vi "Waterfall Page.vi"() -> ()   [LabVIEW 2017, in "3D Waterfall.lvclass"]
uses:
  <vilib>/Math Plots/3D Math Plots/3D Waterfall/3D Waterfall/3D Waterfall.lvclass
  <vilib>/Math Plots/3D Math Plots/3D Waterfall/3D Waterfall/Typedef/3D Waterfall Propery Array.ctl
  <vilib>/Math Plots/3D Math Plots/3D Waterfall/3D Waterfall/Typedef/3D Waterfall Property.ctl
  <vilib>/Math Plots/3D Math Plots/3D Plot/3D Plot/Typedef/Line Type.ctl
  <vilib>/Math Plots/3D Math Plots/3D Plot/3D Plot/Typedef/Color Ramp Cluster.ctl
  <vilib>/Math Plots/3D Math Plots/3D Plot/3D Plot/Typedef/Dialog State.ctl
  <vilib>/Math Plots/3D Math Plots/3D Plot/3D Plot/Typedef/Temp Scene State.ctl
  <vilib>/Math Plots/3D Math Plots/3D Plot/3D Plot/Typedef/Temp Scene Property Action.ctl
  <vilib>/Math Plots/3D Math Plots/3D Plot/3D Plot/3D Plot.lvclass
panel:
  in  "Waterfall Mode":u16(ring) caption="Waterfall mode" items=["Lines", "Slices"]
  in  "Line Style":u16(ring) caption="Line style"
  in  "Antialiasing":bool
  in  "Line Width":sgl=0.001 caption="Line width" min=0.001 step=1
  out "Waterfall Property Out":T1
  in  "Waterfall Property In":T1
  out "Color Ramp":dbl[][](graph)
  in  "Color Map Style":u16(ring) caption="Color map style" items=["None ", "Shaded", "Color spectrum", "Grey scale", "Custom"]
  in  "YZ Plane Projection":bool caption="YZ plane projection"
  in  "XZ Plane Projection":bool caption="XZ plane projection"
  in  "XY Plane Projection":bool caption="XY plane projection"
  in  "Coordinate System":u16(ring) caption="Coordinate system" items=["Cartesian", "Cylindrical", "Spherical"]
  in  "Plot Opacity":sgl(slide) caption="Plot opacity(%)" min=0 max=100 scale=0.0..100.0
  in  "Plot List":i32(listbox)
  in  "Ramp Edit":bool caption="Ramp edit"
  in  "Move Down":bool
  in  "Move Up":bool
  in  "Delete":bool
  in  "New":bool
  in  "Event Registration":refnum<event-registration>
  # "Waterfall"
  # "General"
  # "Projection"
  # "Color Ramp"
  # "Waterfall"
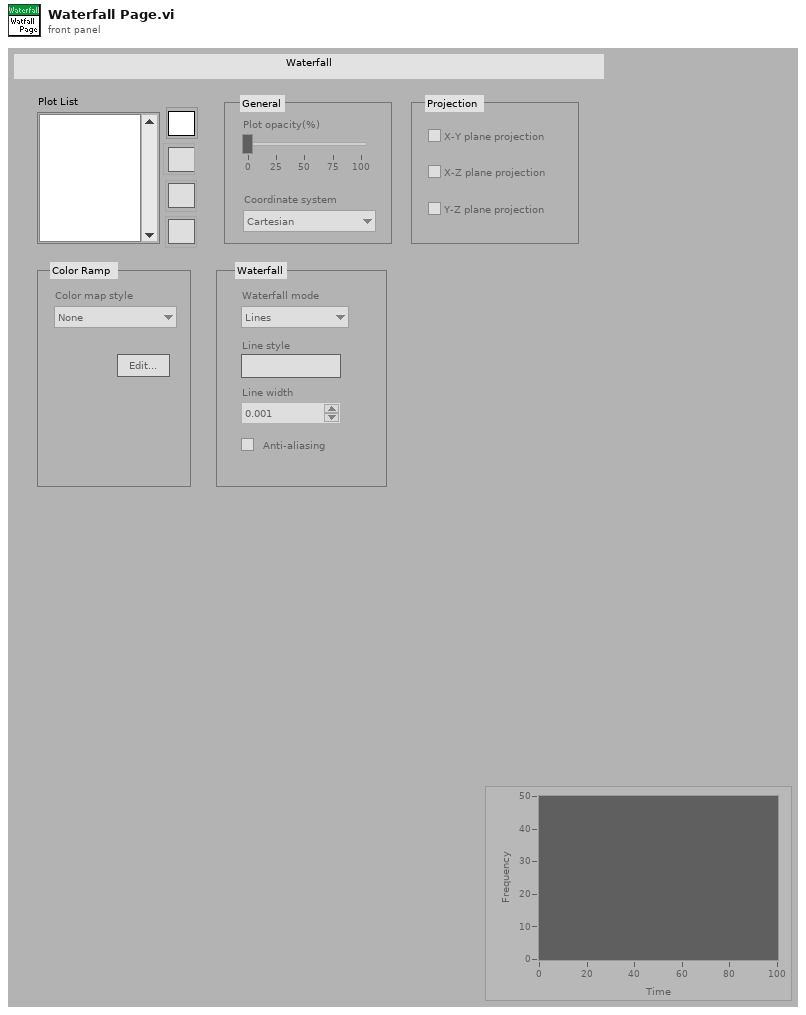
[diagram p1: front panel]
types:
  T1 = typedef "3D Waterfall.lvclass/3D Waterfall Propery Array.ctl" = T2[]
  T2 = typedef "3D Waterfall.lvclass/3D Waterfall Property.ctl" = cluster{"General Property":cluster{"Plot Name":string, "Coordinate System":enum16{"Cartesian", "Cylindrical", "Spherical"}, "Opacity":sgl}, "Projection Property":cluster{"Draw XY":bool, "Draw YZ":bool, "Draw XZ":bool}, "Plot Property":cluster{"Line Style":T3, "Line Width":sgl, "Color Ramp Cluster":T4, "Antialiasing":bool}, "Waterfall Property":cluster{"Waterfall Mode":enum16{"Lines", "Slices"}}}
  T3 = typedef "3D Plot.lvclass/Line Type.ctl" = enum16{"None", "Solid", "Dash", "Dot", "Dash Dot"}
  T4 = typedef "3D Plot.lvclass/Color Ramp Cluster.ctl" = cluster{"Color Ramp Style":enum16{"None", "Shaded", "Color spectrum", "Grey scale", "Custom"}, "Color Ramp Array":u32[], "Color Ramp Index":i32[], "Interpolate?":bool, "Logarithm?":bool}
  T5 = typedef "3D Plot.lvclass/Dialog State.ctl" = enum16{"Initialize", "Read Porperty", "Write Property", "Idle", "Exit"}
  T6 = typedef "3D Plot.lvclass/Temp Scene State.ctl" = enum16{"Create", "Update Scene", "Get Plot Representation", "Destory"}
  T7 = typedef "3D Plot.lvclass/Temp Scene Property Action.ctl" = enum16{"Graph Property", "Light Property", "Axis Property", "Value Pair Property", "Format Property", "Cursor Property", "Plot Specific Property"}
  T8 = typedef "3D Plot.lvclass/Multiplot Representation.ctl" = cluster{"Plot Represention Array":T9[], "Max Range":T10}
  T9 = typedef "3D Plot.lvclass/Plot Representation.ctl" = cluster{"Plot ID":i32, "Plot Range":T10, "Mesh Data":T11, "Dimension":cluster{"X Dimension":i32, "Y Dimension":i32}, "Ramp Range":T10}
  T10 = typedef "3D Plot.lvclass/Range Clusters.ctl" = cluster{"X Range":cluster{"Max X":sgl, "Min X":sgl}, "Y Range":cluster{"Max Y":sgl, "Min Y":sgl}, "Z Range":cluster{"Max Z":sgl, "Min Z":sgl}}
  T11 = typedef "3D Plot.lvclass/Mesh Data.ctl" = cluster{"Index Array":u32[], "Vertex Array":cluster{"X":sgl, "Y":sgl, "Z":sgl}[], "Normal Array":cluster{"X":sgl, "Y":sgl, "Z":sgl}[], "Color Index Array":i32[]}
  T12 = enum16{"None", "Shaded", "Color spectrum", "Grey scale", "Custom"}
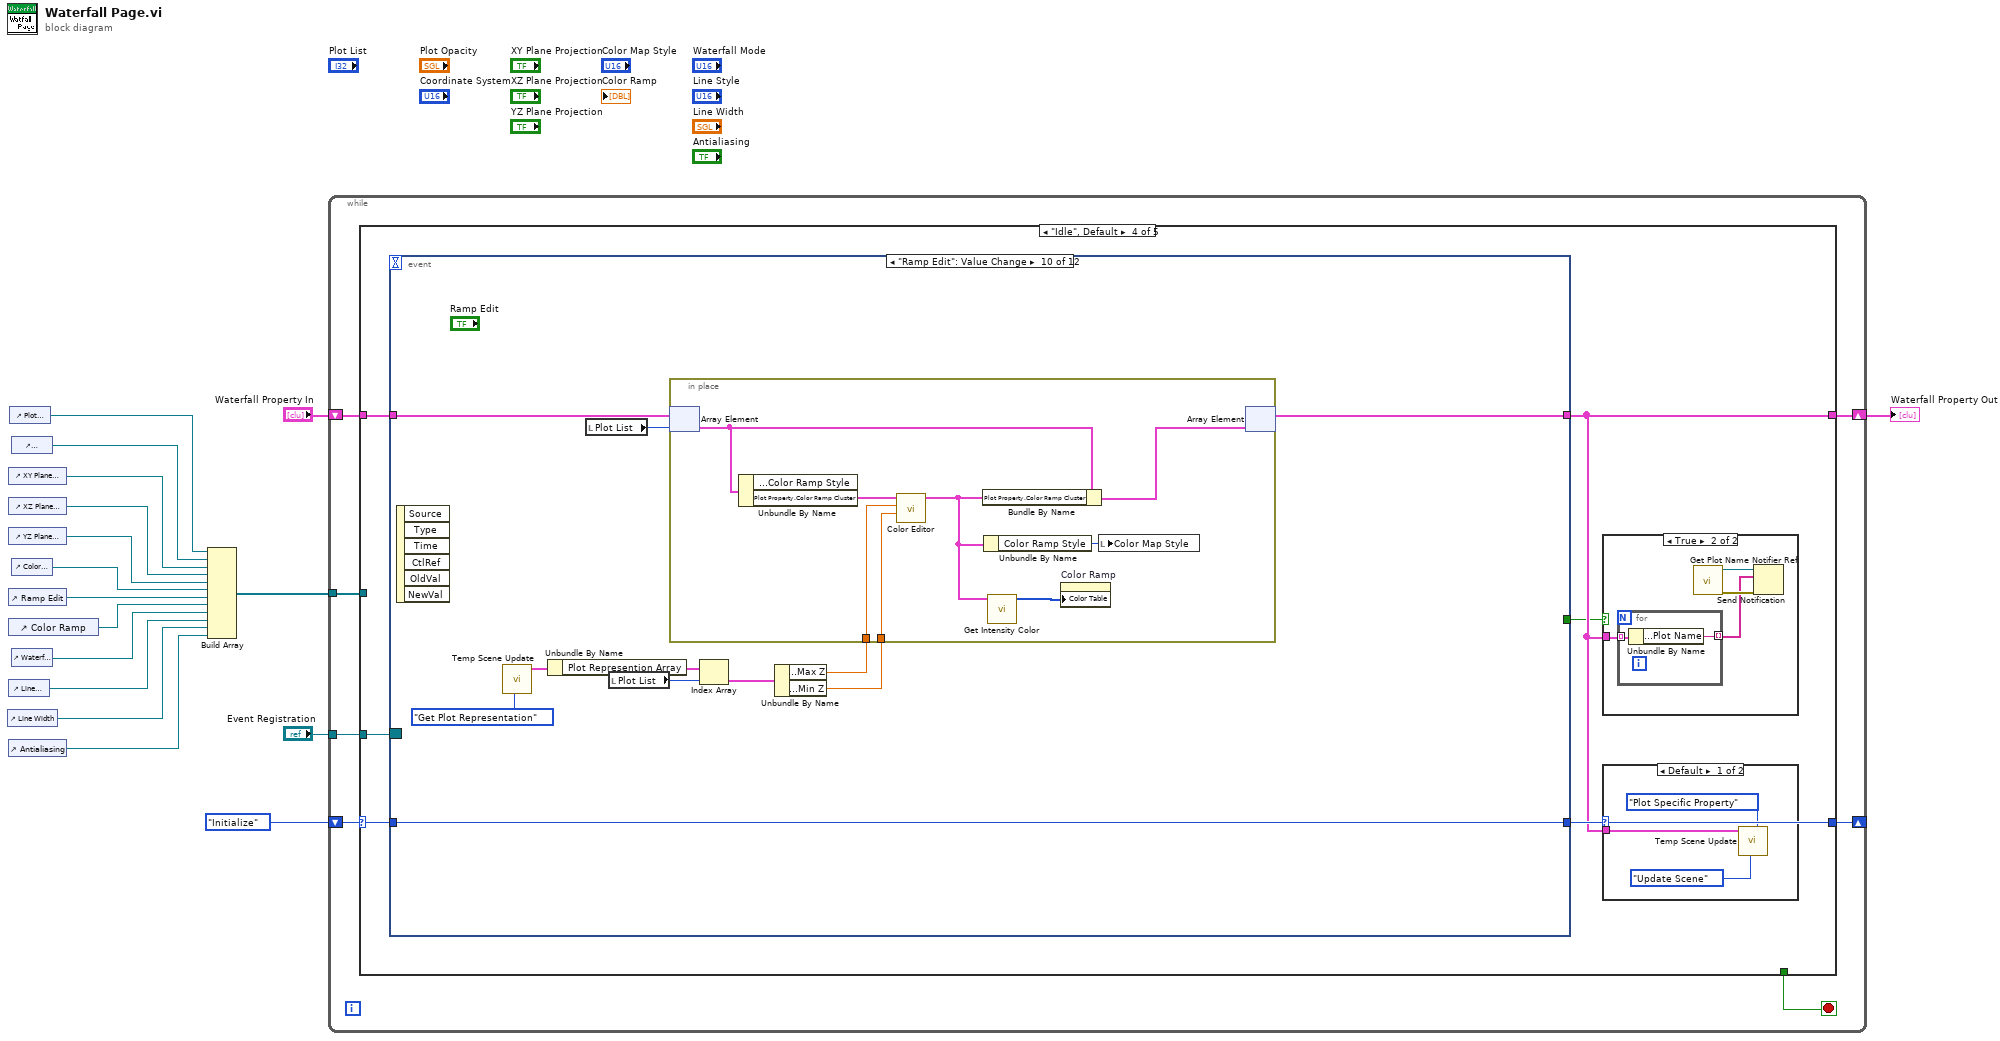
[diagram p0: block diagram]
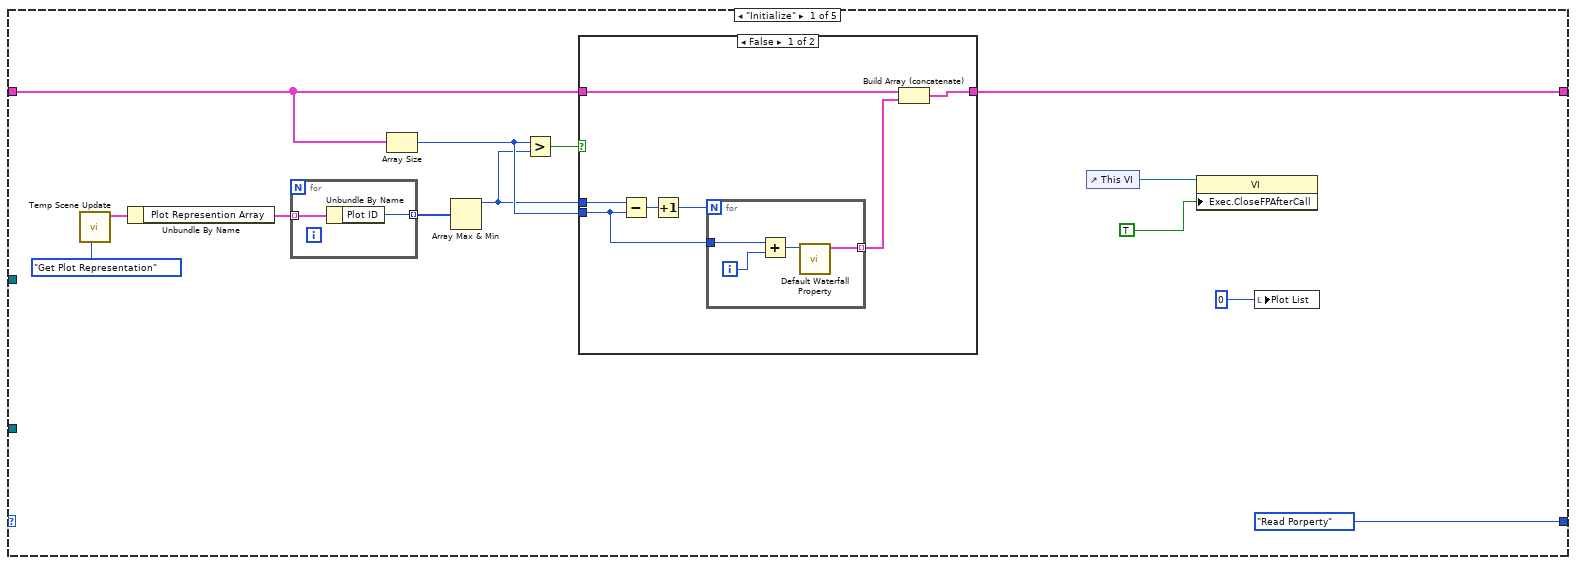
[diagram p2: hidden frame]
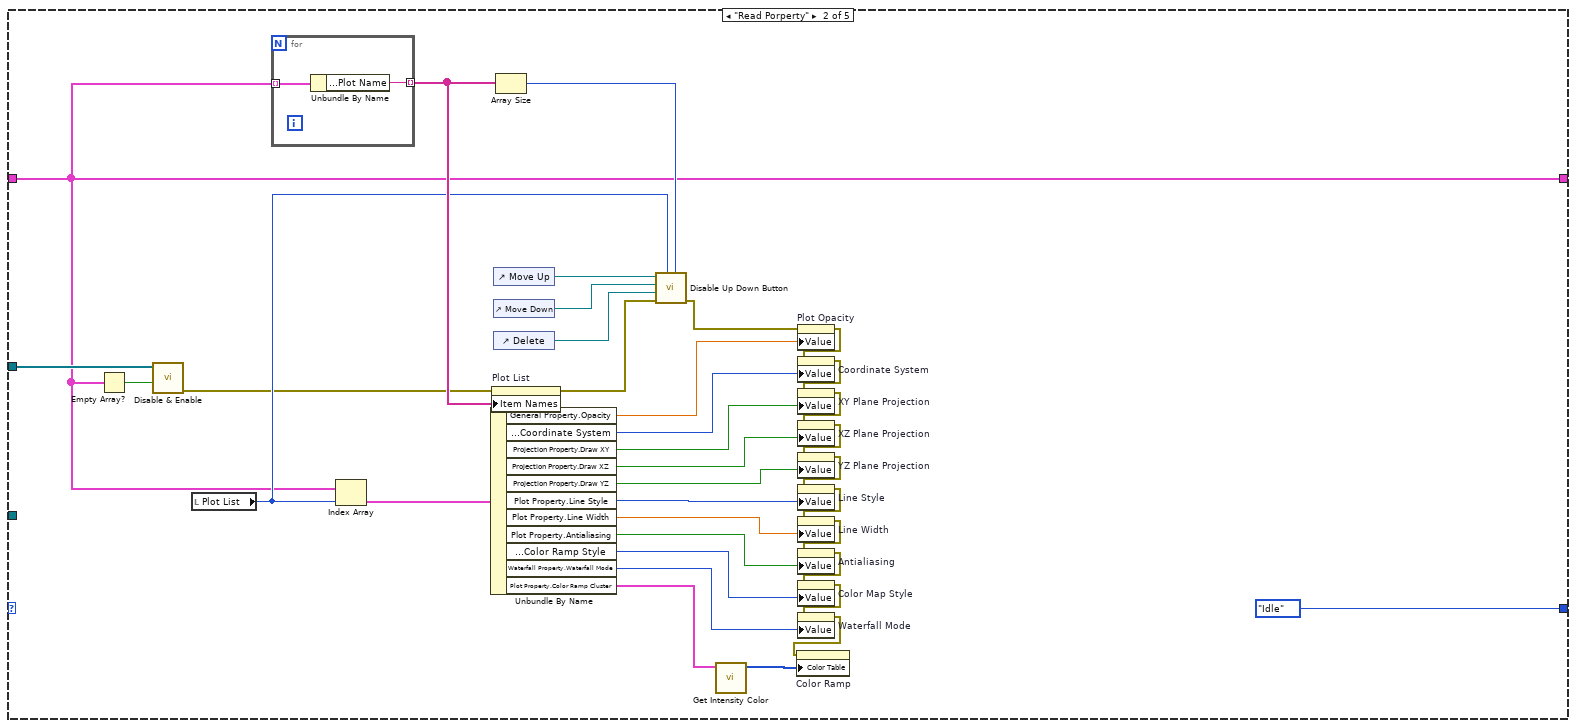
[diagram p4: hidden frame]
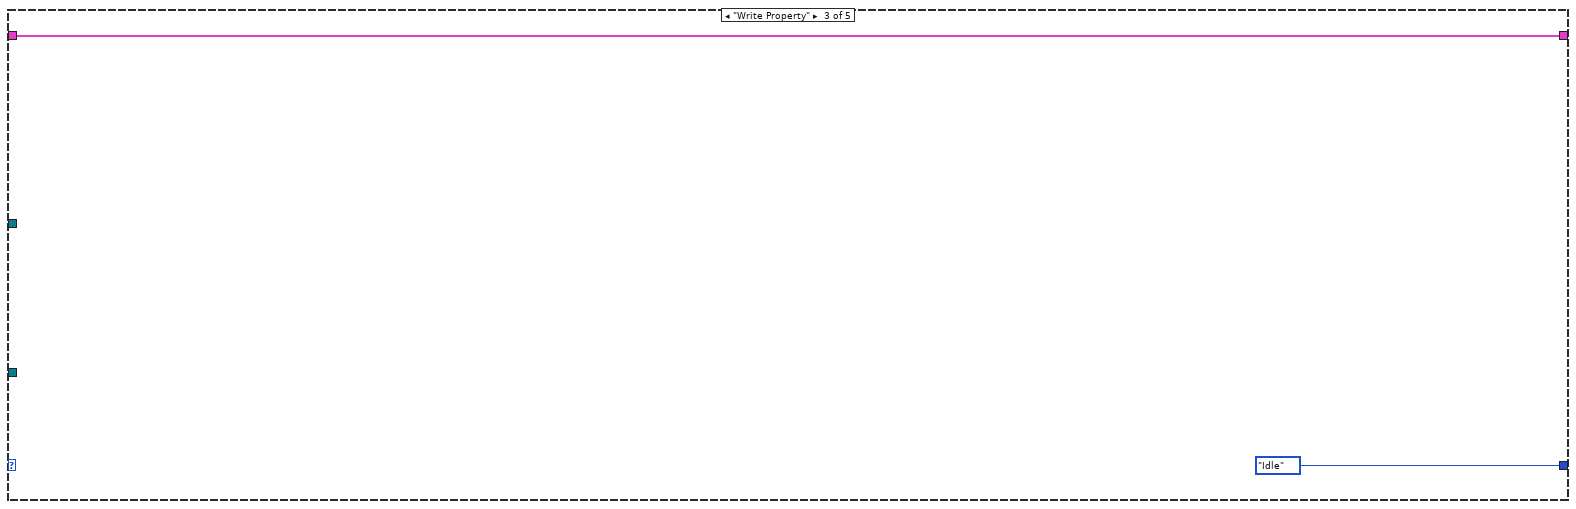
[diagram p5: hidden frame]
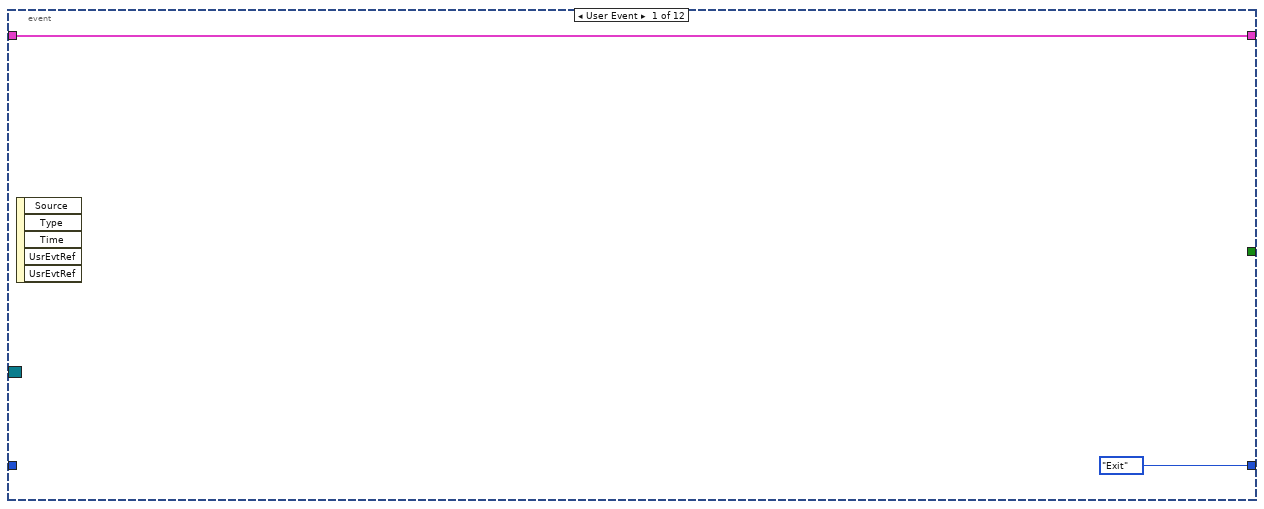
[diagram p8: hidden frame]
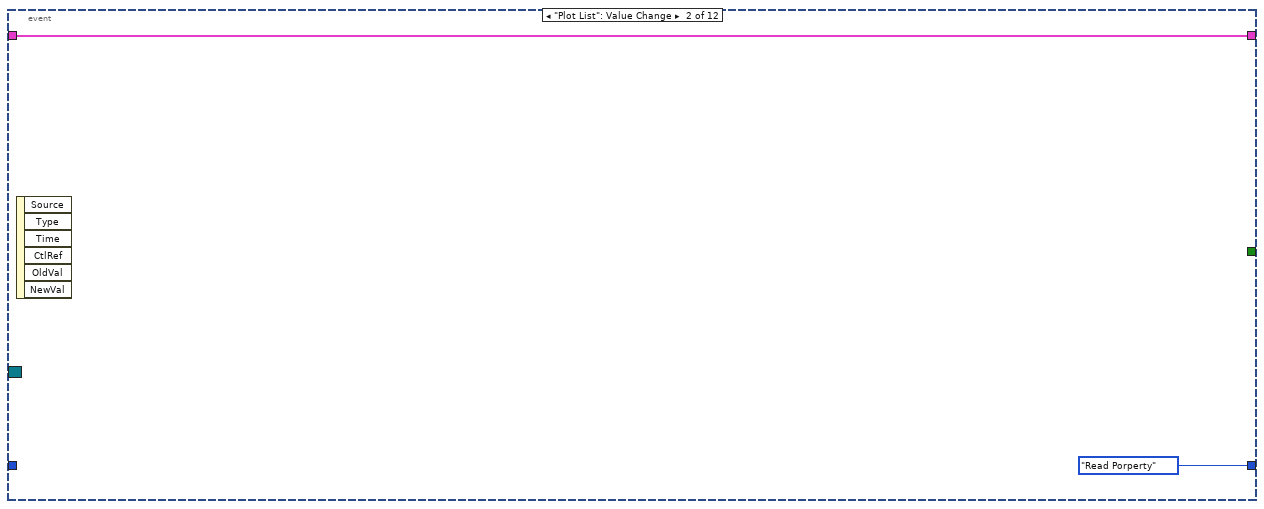
[diagram p9: hidden frame]
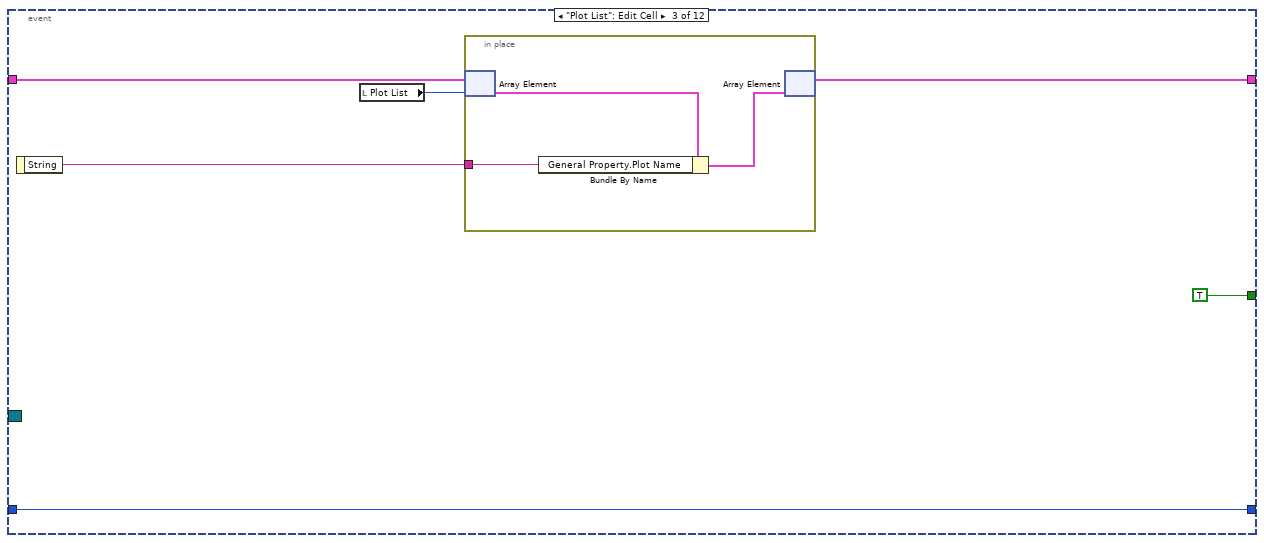
[diagram p10: hidden frame]
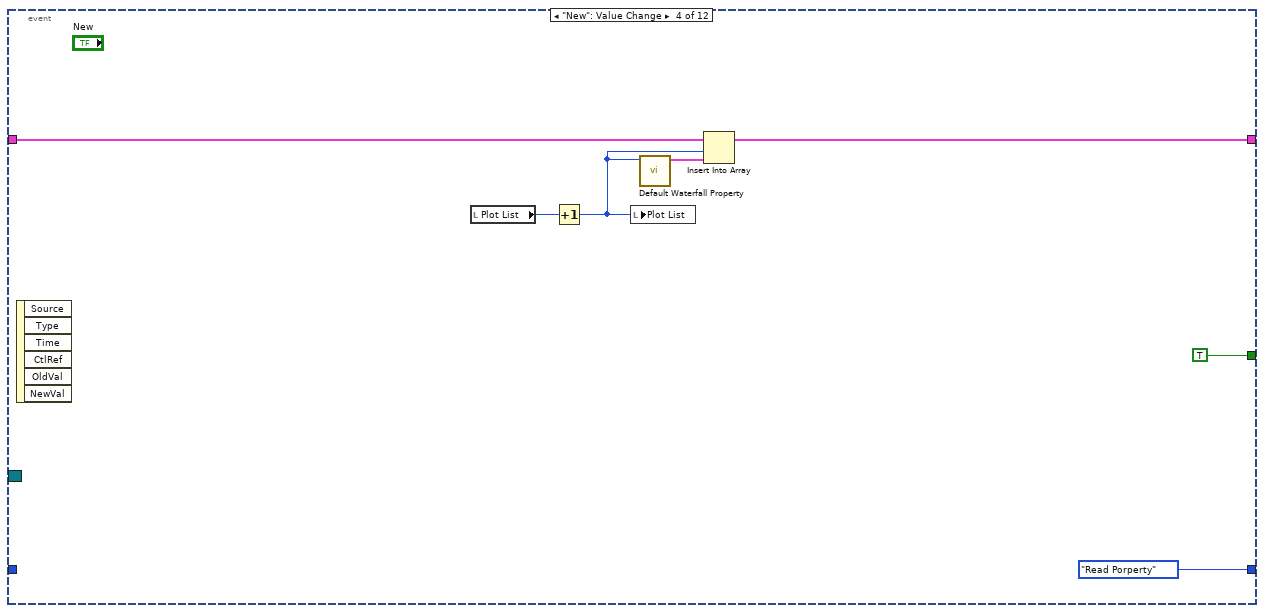
[diagram p11: hidden frame]
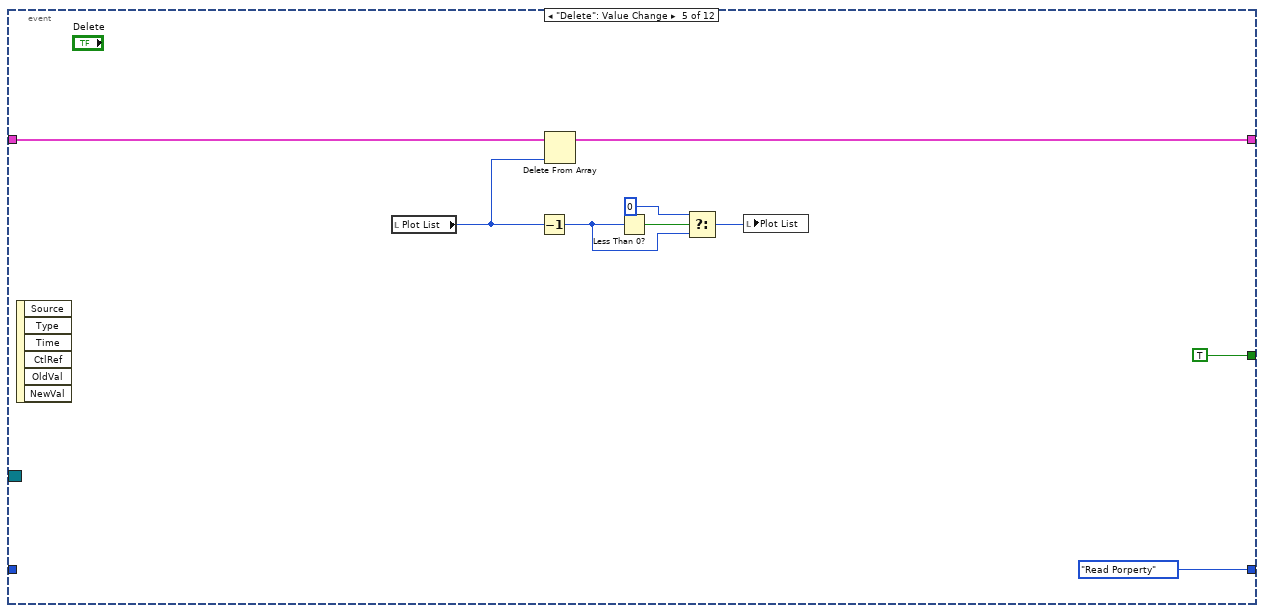
[diagram p12: hidden frame]
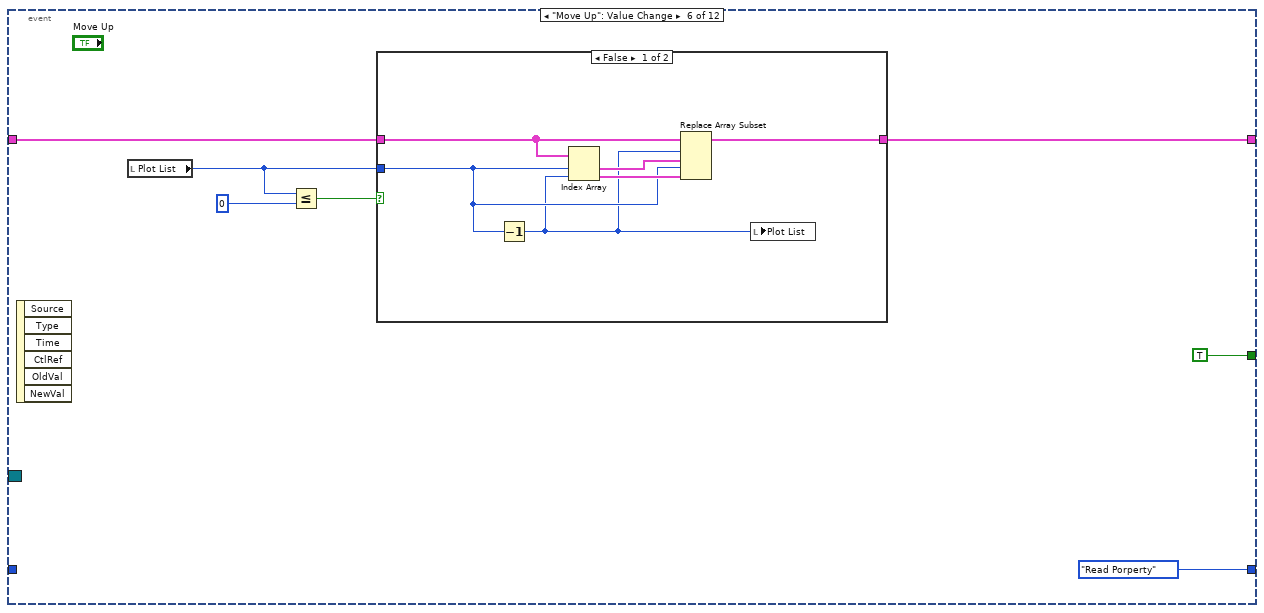
[diagram p13: hidden frame]
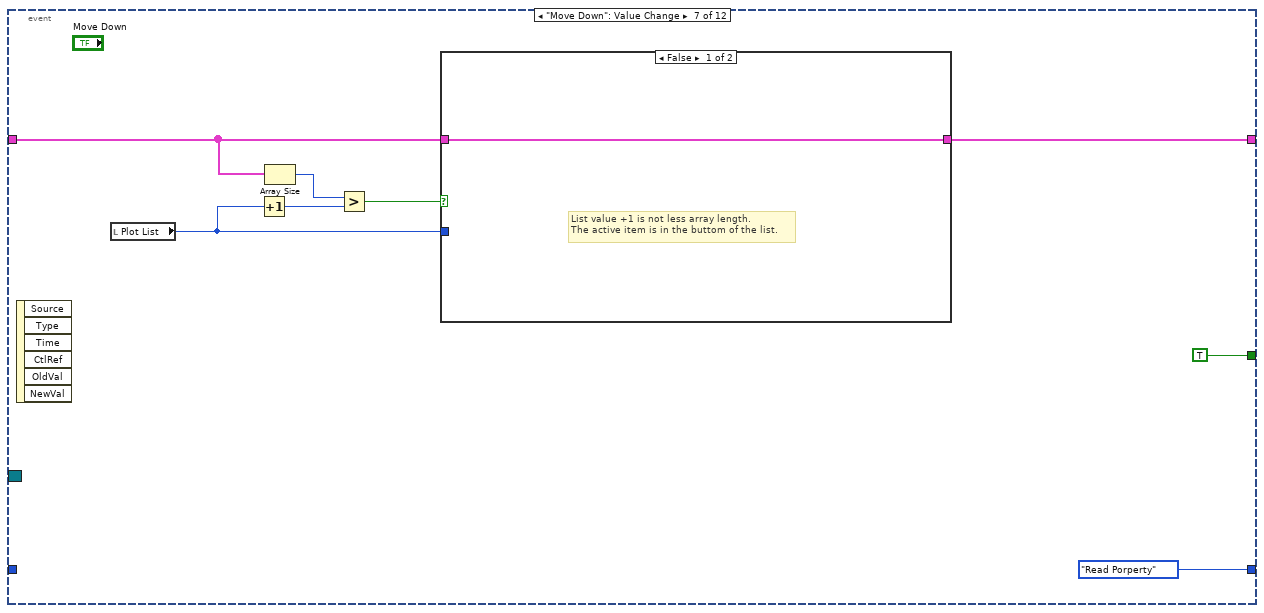
[diagram p15: hidden frame]
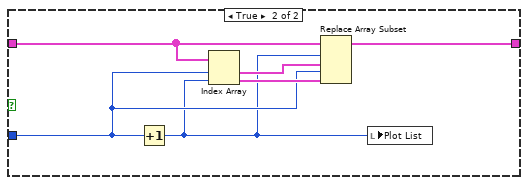
[diagram p16: hidden frame]
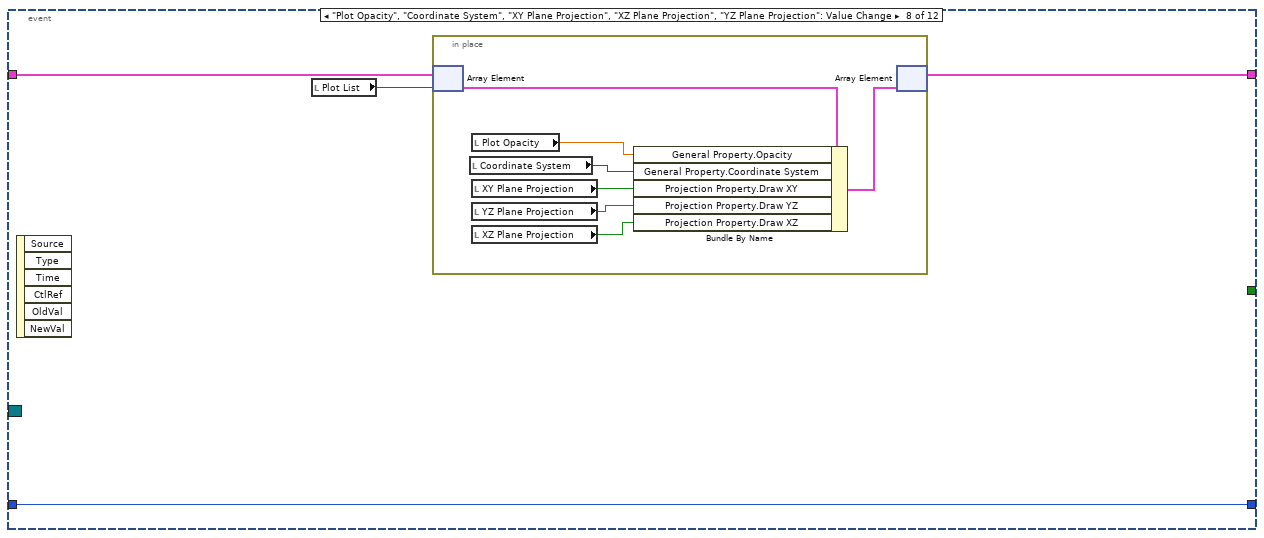
[diagram p17: hidden frame]
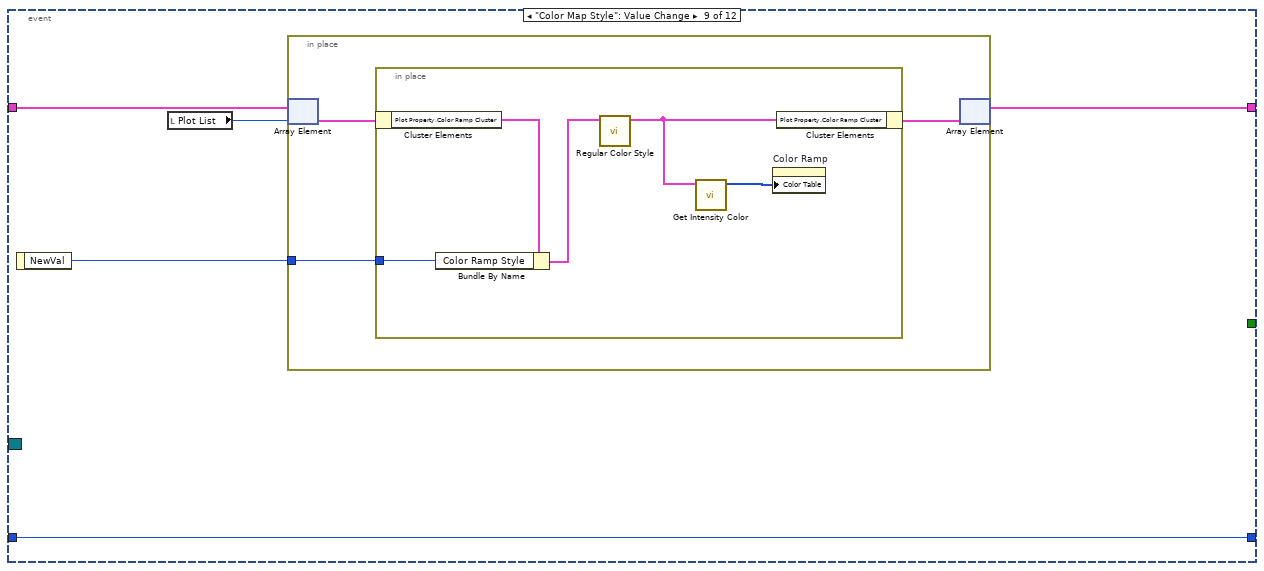
[diagram p18: hidden frame]
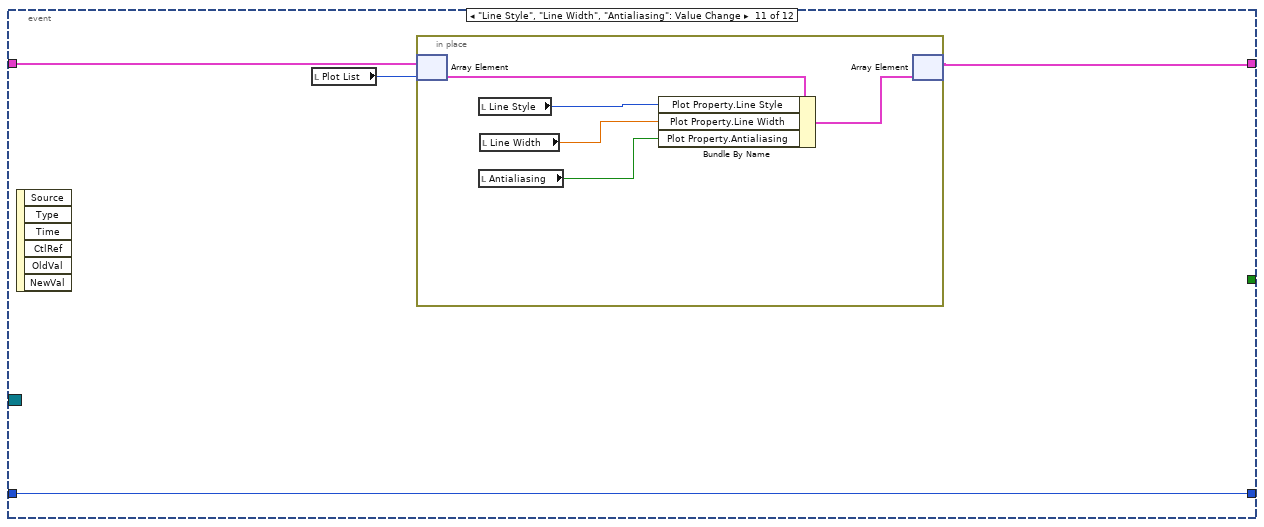
[diagram p19: hidden frame]
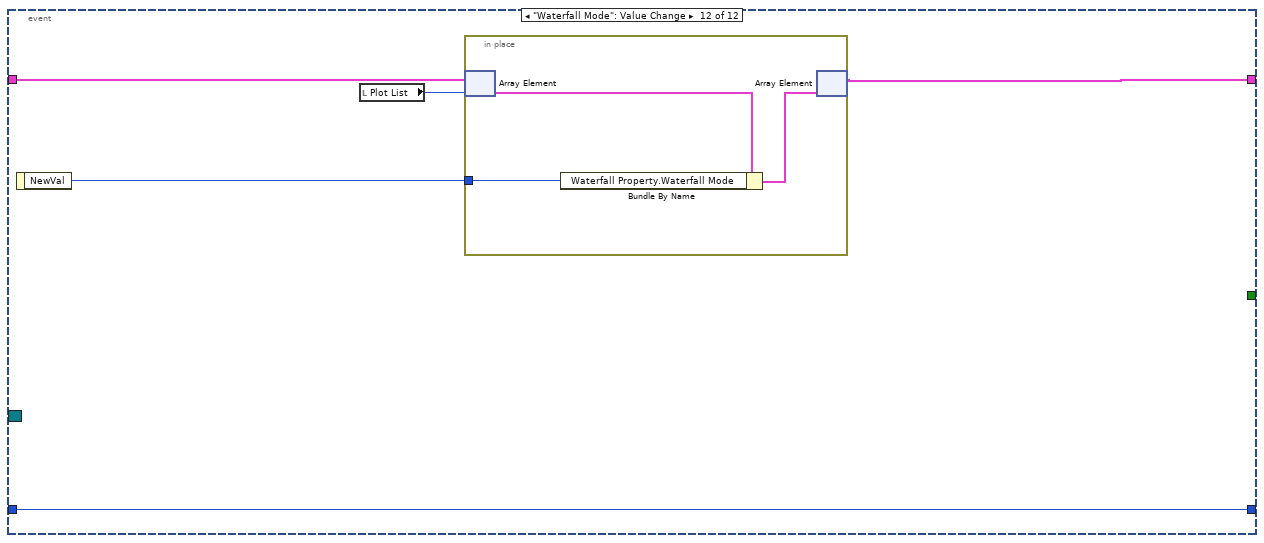
[diagram p20: hidden frame]
diagram:
  n1 = control-ref of="Line Width"() -> (w3:refnum<vi>)
  n2 = control-ref of="XY Plane Projection"() -> (w11:refnum<vi>)
  n3 = control-ref of="XZ Plane Projection"() -> (w10:refnum<vi>)
  n4 = control-ref of="YZ Plane Projection"() -> (w9:refnum<vi>)
  n5 = control-ref of="Ramp Edit"() -> (w7:refnum<vi>)
  n6 = control-ref of="Color Ramp"() -> (w6:refnum<vi>)
  n7 = control-ref of="Line Style"() -> (w4:refnum<vi>)
  n8 = control-ref of="Antialiasing"() -> (w2:refnum<vi>)
  n9 = control-ref of="Plot Opacity"() -> (w13:refnum<vi>)
  n10 = control-ref of="Coordinate System"() -> (w12:refnum<vi>)
  n11 = control-ref of="Color Map Style"() -> (w8:refnum<vi>)
  n12 = control-ref of="Waterfall Mode"() -> (w5:refnum<vi>)
  n13 = Build Array(w13, w12, w11, w10, w9, w8, w7, w6, w5, w4, w3, w2) -> (w1:refnum<vi>[])
  n14 = while {
    shift-right: [w23] -> w14
    shift-left: "Waterfall Property In" -> [w24]
    shift-right: [w19] -> _
    shift-left: Dialog_State."Initialize" -> [w22]
    tunnel: "Event Registration" -> [w20]
    tunnel: w1 -> [w18]
    stop <- w21 stop-if-true
    n15 = case shown="\"Idle\", Default" w22 {
      selector: w22 -> [_ _ _ w95 _]
      tunnel: w24 -> [w27 w74 w90 w97 w225]
      tunnel: [w26 w74 w90 w93 w225] -> w23
      tunnel: [Dialog_State."Read Porperty" Dialog_State."Idle" Dialog_State."Idle" w94 Dialog_State."Exit"] -> w19
      tunnel: [_ _ _ _ TRUE] -> w21
      tunnel: w20 -> [_ _ _ w96 _]
      tunnel: w18 -> [_ w76 _ _ _]
      frame "Initialize" {
        n16 = call <vilib>:"Temp Scene Update.vi"("State"=Temp_Scene_State."Get Plot Representation") -> ("Multiplot Representation"=w32:T8)  [unwired: 5 in, 5 out]
        n17 = Unbundle By Name(w32) -> ("Plot Represention Array"=w25:T9[])
        n18 = for {
          tunnel: w25 -> [w51] mode=indexing
          tunnel: [w50] -> w31 mode=indexing
          n19 = Unbundle By Name(w51) -> ("Plot ID"=w50:i32)
        }
        n20 = Array Size(array=w27) -> (size(s)=w29:i32)
        n21 = Array Max & Min(array=w31) -> (max value=w28:i32)  [unwired: 3 out]
        n22 = Greater?(x=w29, y=w28) -> (0:w30:bool)
        n23 = case shown="False" w30 {
          tunnel: [w42 w49] -> w26
          tunnel: w27 -> [w44 w49]
          tunnel: w29 -> [w38 _]
          tunnel: w28 -> [w39 _]
          frame False {
            n24 = Subtract(x=w39, y=w38) -> (x-y=w41:i32)
            n25 = Increment(x=w41) -> (x+1=w40:i32)
            n26 = for {
              N: w40 -> [_]
              tunnel: w38 -> [w47]
              tunnel: [w45] -> w43 mode=indexing
              i -> [w48]
              n27 = Add(x=w47, y=w48) -> (x+y=w46:i32)
              n28 = call <vilib>:"Default Waterfall Property.vi"("Plot ID"=w46) -> ("Default Property"=w45:T2)  [unwired: 10 out]
            }
            n29 = Build Array (concatenate)(w44, w43) -> (w42:T1)
          }
          frame True {
          }
        }
        n30 = control-ref of="This VI"() -> (w36:refnum<vi>)
        n31 = property class="VI"(reference=w36, "Exec.CloseFPAfterCall"=TRUE ("Execution:Close After Call")) -> ()  [unwired: 1 in, 2 out]
        n32 = local write "Plot List"(0 ("Plot List")) -> ()
      }
      frame "Read Porperty" {
        n33 = Empty Array?(array=w74) -> (empty?=w75:bool)
        n34 = call <vilib>:"Disable & Enable.vi"("Disabled?"=w75, "Control Ref Array"=w76) -> ("error out"=w73:errorcluster)  [unwired: 1 in, 8 out]
        n35 = local read "Plot List"() -> (w77:i32)
        n36 = for {
          tunnel: w74 -> [w89] mode=indexing
          tunnel: [w88] -> w79 mode=indexing
          n37 = Unbundle By Name(w89) -> ("General Property.Plot Name"=w88:string)
        }
        n38 = Index Array(array=w74, index=w77) -> (element=w86:T2)
        n39 = Unbundle By Name(w86) -> ("General Property.Opacity"=w72:sgl, "General Property.Coordinate System"=w71:enum16{"Cartesian", "Cylindrical", "Spherical"}, "Projection Property.Draw XY"=w70:bool, "Projection Property.Draw XZ"=w69:bool, "Projection Property.Draw YZ"=w68:bool, "Plot Property.Line Style"=w67:T3, "Plot Property.Line Width"=w66:sgl, "Plot Property.Antialiasing"=w65:bool, "Plot Property.Color Ramp Cluster.Color Ramp Style"=w63:T12, "Waterfall Property.Waterfall Mode"=w64:enum16{"Lines", "Slices"}, "Plot Property.Color Ramp Cluster"=w85:T4)
        n40 = property on="Plot List" class="LstBox (strict)"(error in=w73, "Item Names"=w79) -> (error out=w78:errorcluster)  [unwired: 1 in, 1 out]
        n41 = control-ref of="Move Up"() -> (w81:refnum<vi>)
        n42 = control-ref of="Move Down"() -> (w82:refnum<vi>)
        n43 = control-ref of="Delete"() -> (w83:refnum<vi>)
        n44 = Array Size(array=w79) -> (size(s)=w80:i32)
        n45 = call <vilib>:"Disable Up Down Button.vi"("Length"=w80, "Index"=w77, "error in (no error)"=w78, "Delete Ref"=w83, "Move Down Ref"=w82, "Move Up Ref"=w81) -> ("error out"=w62:errorcluster)  [unwired: 5 out]
        n46 = call <vilib>:"Get Intensity Color.vi"("Color Ramp Cluster"=w85) -> ("Intensity Color"=w84:u32[])  [unwired: 4 in, 6 out]
        n47 = property on="Plot Opacity" class="Slide (strict)"(error in=w62, "Value"=w72) -> (error out=w61:errorcluster)  [unwired: 1 in, 1 out]
        n48 = property on="Coordinate System" class="Ring (strict)"(error in=w61, "Value"=w71) -> (error out=w60:errorcluster)  [unwired: 1 in, 1 out]
        n49 = property on="XY Plane Projection" class="Bool (strict)"(error in=w60, "Value"=w70) -> (error out=w59:errorcluster)  [unwired: 1 in, 1 out]
        n50 = property on="XZ Plane Projection" class="Bool (strict)"(error in=w59, "Value"=w69) -> (error out=w58:errorcluster)  [unwired: 1 in, 1 out]
        n51 = property on="YZ Plane Projection" class="Bool (strict)"(error in=w58, "Value"=w68) -> (error out=w57:errorcluster)  [unwired: 1 in, 1 out]
        n52 = property on="Line Style" class="Ring (strict)"(error in=w57, "Value"=w67) -> (error out=w56:errorcluster)  [unwired: 1 in, 1 out]
        n53 = property on="Line Width" class="DigNum (strict)"(error in=w56, "Value"=w66) -> (error out=w55:errorcluster)  [unwired: 1 in, 1 out]
        n54 = property on="Antialiasing" class="Bool (strict)"(error in=w55, "Value"=w65) -> (error out=w54:errorcluster)  [unwired: 1 in, 1 out]
        n55 = property on="Color Map Style" class="Ring (strict)"(error in=w54, "Value"=w63) -> (error out=w53:errorcluster)  [unwired: 1 in, 1 out]
        n56 = property on="Waterfall Mode" class="Ring (strict)"(error in=w53, "Value"=w64) -> (error out=w52:errorcluster)  [unwired: 1 in, 1 out]
        n57 = property on="Color Ramp" class="IntGraph (strict)"(error in=w52, "Color Table"=w84) -> ()  [unwired: 1 in, 2 out]
      }
      frame "Write Property" {
      }
      frame "Idle", Default {
        n58 = event shown="[9] \"Ramp Edit\": Value Change" {
          selector: w96 -> [_ _ _ _ _ _ _ _ _ _ _ _]
          dyn-events: _ -> [_ _ _ _ _ _ _ _ _ _ _ _]
          timeout: _ -> [_ _ _ _ _ _ _ _ _ _ _ _]
          tunnel: w97 -> [w108 w110 w114 w124 w133 w138 w152 w166 w179 w197 w209 w219]
          tunnel: [w108 w110 w113 w123 w134 w137 w151 w165 w176 w196 w208 w218] -> w93
          tunnel: [Dialog_State."Exit" Dialog_State."Read Porperty" w112 Dialog_State."Read Porperty" Dialog_State."Read Porperty" Dialog_State."Read Porperty" Dialog_State."Read Porperty" w168 w180 w199 w211 w220] -> w94
          tunnel: w95 -> [_ _ w112 _ _ _ _ w168 w180 w199 w211 w220]
          tunnel: [_ _ TRUE TRUE TRUE TRUE TRUE _ _ _ _ _] -> w92
          event User Event {
            n59 = event-data() -> ()  [unwired: 6 out]
          }
          event "Plot List": Value Change {
            n60 = event-data() -> ()  [unwired: 7 out]
          }
          event "Plot List": Edit Cell {
            n61 = event-data() -> ("String"=w115:string)  [unwired: 1 out]
            n62 = local read "Plot List"() -> (w116:i32)
            n63 = in-place {
              in-place-border: w115 -> [w117]
              n64 = in-place-array #1(w114, w116) -> (w119:T2)
              n65 = Bundle By Name(cluster=w119, "General Property.Plot Name"=w117) -> (w118:T2)
              n66 = in-place-array #1(w118) -> (w113:T1)  [unwired: 1 out]
            }
          }
          event "New": Value Change {
            n67 = event-data() -> ()  [unwired: 7 out]
            n68 = local read "Plot List"() -> (w125:i32)
            n69 = Increment(x=w125) -> (x+1=w121:i32)
            n70 = local write "Plot List"(w121) -> ()
            n71 = call <vilib>:"Default Waterfall Property.vi"("Plot ID"=w121) -> ("Default Property"=w120:T2)  [unwired: 10 out]
            n72 = Insert Into Array(array=w124, index=w121, new element=w120) -> (w123:T1)
          }
          event "Delete": Value Change {
            n73 = event-data() -> ()  [unwired: 7 out]
            n74 = local read "Plot List"() -> (w129:i32)
            n75 = Decrement(x=w129) -> (x-1=w130:i32)
            n76 = Delete From Array(array=w133, index=w129) -> (array with subset deleted=w134:T1)  [unwired: 1 in, 1 out]
            n77 = Less Than 0?(x=w130) -> (x < 0?=w132:bool)
            n78 = Select(t=0, s=w132, f=w130) -> (s? t:f=w128:i32)
            n79 = local write "Plot List"(w128) -> ()
          }
          event "Move Up": Value Change {
            n80 = event-data() -> ()  [unwired: 7 out]
            n81 = local read "Plot List"() -> (w139:i32)
            n82 = Less Or Equal?(x=w139, y=0) -> (x <= y?=w141:bool)
            n83 = case shown="False" w141 {
              tunnel: w138 -> [w146 w149]
              tunnel: [w145 w149] -> w137
              tunnel: w139 -> [w144 _]
              frame False {
                n84 = Decrement(x=w144) -> (x-1=w143:i32)
                n85 = Index Array(array=w146, index #1=w144, index #2=w143) -> (element #1=w148:T2, element #2=w147:T2)
                n86 = Replace Array Subset(array=w146, new element #1=w148, index #1=w143, new element #2=w147, index #2=w144) -> (w145:T1)
                n87 = local write "Plot List"(w143) -> ()
              }
              frame True {
                # "List value is less or equal to 0.\nThe active item is in the top of the list."
              }
            }
          }
          event "Move Down": Value Change {
            n88 = event-data() -> ()  [unwired: 7 out]
            n89 = local read "Plot List"() -> (w153:i32)
            n90 = Increment(x=w153) -> (x+1=w155:i32)
            n91 = Array Size(array=w152) -> (size(s)=w156:i32)
            n92 = Greater?(x=w156, y=w155) -> (0:w154:bool)
            n93 = case shown="False" w154 {
              tunnel: w152 -> [w158 w162]
              tunnel: [w158 w161] -> w151
              tunnel: w153 -> [_ w160]
              frame False {
                # "List value +1 is not less array length.\nThe active item is in the buttom of the list."
              }
              frame True {
                n94 = Increment(x=w160) -> (x+1=w159:i32)
                n95 = Index Array(array=w162, index #1=w160, index #2=w159) -> (element #1=w164:T2, element #2=w163:T2)
                n96 = Replace Array Subset(array=w162, new element #1=w164, index #1=w159, new element #2=w163, index #2=w160) -> (w161:T1)
                n97 = local write "Plot List"(w159) -> ()
              }
            }
          }
          event "Plot Opacity", "Coordinate System", "XY Plane Projection", "XZ Plane Projection", "YZ Plane Projection": Value Change {
            n98 = event-data() -> ()  [unwired: 7 out]
            n99 = local read "Plot List"() -> (w167:i32)
            n100 = in-place {
              n101 = in-place-array #2(w166, w167) -> (w171:T2)
              n102 = local read "Coordinate System"() -> (w169:u16)
              n103 = local read "Plot Opacity"() -> (w175:sgl)
              n104 = local read "XY Plane Projection"() -> (w174:bool)
              n105 = local read "YZ Plane Projection"() -> (w172:bool)
              n106 = local read "XZ Plane Projection"() -> (w173:bool)
              n107 = Bundle By Name(cluster=w171, "General Property.Opacity"=w175, "General Property.Coordinate System"=w169, "Projection Property.Draw XY"=w174, "Projection Property.Draw YZ"=w172, "Projection Property.Draw XZ"=w173) -> (w170:T2)
              n108 = in-place-array #2(w170) -> (w165:T1)  [unwired: 1 out]
            }
          }
          event "Color Map Style": Value Change {
            n109 = event-data() -> ("NewVal"=w177:u16)  [unwired: 1 out]
            n110 = local read "Plot List"() -> (w178:i32)
            n111 = in-place {
              in-place-border: w177 -> [w182]
              n112 = in-place-array #3(w179, w178) -> (w183:T2)
              n113 = in-place {
                in-place-border: w182 -> [w187]
                n114 = in-place-cluster #4(w183) -> ("Plot Property.Color Ramp Cluster"=w188:T4)
                n115 = Bundle By Name(cluster=w188, "Color Ramp Style"=w187) -> (w186:T4)
                n116 = call <vilib>:"Regular Color Style.vi"("Color Ramp Cluster in"=w186) -> ("Color Ramp Cluster out"=w184:T4)  [unwired: 10 in]
                n117 = call <vilib>:"Get Intensity Color.vi"("Color Ramp Cluster"=w184) -> ("Intensity Color"=w185:u32[])  [unwired: 4 in, 6 out]
                n118 = property on="Color Ramp" class="IntGraph (strict)"("Color Table"=w185) -> ()  [unwired: 2 in, 2 out]
                n119 = in-place-cluster #4("Plot Property.Color Ramp Cluster"=w184) -> (w181:T2)
              }
              n120 = in-place-array #3(w181) -> (w176:T1)  [unwired: 1 out]
            }
          }
          event "Ramp Edit": Value Change {
            n121 = event-data() -> ()  [unwired: 7 out]
            n122 = call <vilib>:"Temp Scene Update.vi"("State"=Temp_Scene_State."Get Plot Representation") -> ("Multiplot Representation"=w192:T8)  [unwired: 5 in, 5 out]
            n123 = Unbundle By Name(w192) -> ("Plot Represention Array"=w189:T9[])
            n124 = local read "Plot List"() -> (w198:i32)
            n125 = local read "Plot List"() -> (w195:i32)
            n126 = Index Array(array=w189, index=w195) -> (element=w194:T9)
            n127 = Unbundle By Name(w194) -> ("Plot Range.Z Range.Max Z"=w191:sgl, "Plot Range.Z Range.Min Z"=w190:sgl)
            n128 = in-place {
              in-place-border: w191 -> [w203]
              in-place-border: w190 -> [w202]
              n129 = in-place-array #5(w197, w198) -> (w206:T2)
              n130 = Unbundle By Name(w206) -> ("Plot Property.Color Ramp Cluster"=w205:T4)  [unwired: 1 out]
              n131 = call <vilib>:"Color Editor.vi"("Min"=w202, "Max"=w203, "Color Ramp Cluster in"=w205) -> ("Color Ramp Cluster out"=w201:T4)  [unwired: 3 in, 5 out]
              n132 = Bundle By Name(cluster=w206, "Plot Property.Color Ramp Cluster"=w201) -> (w207:T2)
              n133 = Unbundle By Name(w201) -> ("Color Ramp Style"=w200:T12)
              n134 = call <vilib>:"Get Intensity Color.vi"("Color Ramp Cluster"=w201) -> ("Intensity Color"=w204:u32[])  [unwired: 4 in, 6 out]
              n135 = property on="Color Ramp" class="IntGraph (strict)"("Color Table"=w204) -> ()  [unwired: 2 in, 2 out]
              n136 = local write "Color Map Style"(w200) -> ()
              n137 = in-place-array #5(w207) -> (w196:T1)  [unwired: 1 out]
            }
          }
          event "Line Style", "Line Width", "Antialiasing": Value Change {
            n138 = event-data() -> ()  [unwired: 7 out]
            n139 = local read "Plot List"() -> (w210:i32)
            n140 = in-place {
              n141 = in-place-array #6(w209, w210) -> (w213:T2)
              n142 = local read "Line Style"() -> (w216:u16)
              n143 = local read "Antialiasing"() -> (w214:bool)
              n144 = local read "Line Width"() -> (w215:sgl)
              n145 = Bundle By Name(cluster=w213, "Plot Property.Line Style"=w216, "Plot Property.Line Width"=w215, "Plot Property.Antialiasing"=w214) -> (w212:T2)
              n146 = in-place-array #6(w212) -> (w208:T1)  [unwired: 1 out]
            }
          }
          event "Waterfall Mode": Value Change {
            n147 = event-data() -> ("NewVal"=w217:u16)  [unwired: 1 out]
            n148 = local read "Plot List"() -> (w221:i32)
            n149 = in-place {
              in-place-border: w217 -> [w222]
              n150 = in-place-array #7(w219, w221) -> (w224:T2)
              n151 = Bundle By Name(cluster=w224, "Waterfall Property.Waterfall Mode"=w222) -> (w223:T2)
              n152 = in-place-array #7(w223) -> (w218:T1)  [unwired: 1 out]
            }
          }
        }
        n153 = case shown="True" w92 {
          tunnel: w93 -> [_ w98]
          frame False {
          }
          frame True {
            n154 = for {
              tunnel: w98 -> [w103] mode=indexing
              tunnel: [w102] -> w99 mode=indexing
              n155 = Unbundle By Name(w103) -> ("General Property.Plot Name"=w102:string)
            }
            n156 = call <vilib>:"Get Plot Name Notifier Ref.vi"() -> ("error out"=w101:errorcluster, "Plot Names Notifier Ref"=w100:refnum<notifier>)  [unwired: 1 in, 9 out]
            n157 = Send Notification(notification=w99, notifier=w100, error in (no error)=w101) -> ()  [unwired: 2 out]
          }
        }
        n158 = case shown="Default" w94 {
          tunnel: w93 -> [w106 _]
          frame Default {
            n159 = call <vilib>:"Temp Scene Update.vi"("Property Name"=Temp_Scene_Property_Action."Plot Specific Property", "State"=Temp_Scene_State."Update Scene", "Property In"=w106) -> ()  [unwired: 3 in, 6 out]
          }
          frame "Exit" {
          }
        }
      }
      frame "Exit" {
      }
    }
  }
  "Waterfall Property Out" <- w14
